vi "Generate Error.vi"(11 "Error":i32) -> (0 "error out":errorcluster)   [LabVIEW 2012, in "OpenCLV x64.lvlib"]
doc: "Converts OpenCL errors to Labview sanctioned error codes in the -5000 to -5999 range."
uses:
  OpenCLV x64.lvlib
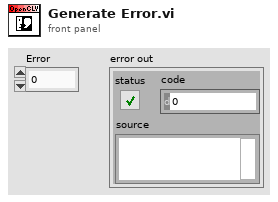
[diagram p1: front panel]
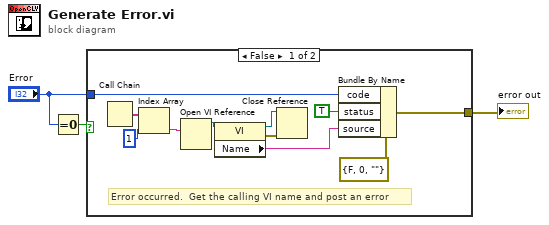
[diagram p0: block diagram]
diagram:
  n1 = Equal To 0?(x="Error") -> (x = 0?=w3:bool)
  n2 = case shown="False" w3 {
    tunnel: "Error" -> [w9 _]
    tunnel: [w7 _] -> w1
    frame False {
      # "Error occurred.  Get the calling VI name and post an error"
      n3 = Call Chain() -> (call chain=w13:string[])
      n4 = Index Array(array=w13, index=1) -> (element=w14:string)
      n5 = Open VI Reference(vi path=w14) -> (vi reference=w11:refnum<vi>)  [unwired: 5 in, 1 out]
      n6 = property class="VI"(reference=w11) -> (reference out=w4:refnum<vi>, error out=w5:errorcluster, "Name"=w12:string)  [unwired: 1 in]
      n7 = Close Reference(reference=w4, error in (no error)=w5) -> ()  [unwired: 1 out]
      n8 = Bundle By Name(cluster=errorcluster {"status"=FALSE, "code"=0, "source"=""} ("error constant"), "code"=w9, "status"=TRUE, "source"=w12) -> (w7:errorcluster)
    }
    frame True {
      # "No Error"
    }
  }
  "error out" <- w1
